vi "Measurement.WavelengthSweeping.GetStaticDependencies.vi"(8 "error in (no error)":errorcluster, 11 "Measurement.WavelengthSweeping in":refnum<class "Measurement.WavelengthSweeping.lvclass">) -> (0 "error out":errorcluster, 2 "Dependencies":T1, 3 "Measurement.WavelengthSweeping out":refnum<class "Measurement.WavelengthSweeping.lvclass">)   [LabVIEW 2019, in "Measurement.WavelengthSweeping.lvclass"]
uses:
  Measurement.WavelengthSweeping.lvclass
  C:/Program Files (x86)/National Instruments/LabVIEW 2019/vi.lib/JKI/JKI SMO/SMO/SMO.lvclass
  Typedefs/Dependencies--Cluster.ctl
  SMU/SMU.lvclass
  LIA/LIA.lvclass
  OPM/OPM.lvclass
  OPA/OPA.lvclass
  MC/MC.lvclass
  <vilib>/JKI/JKI SMO/SMO/SMO.lvclass
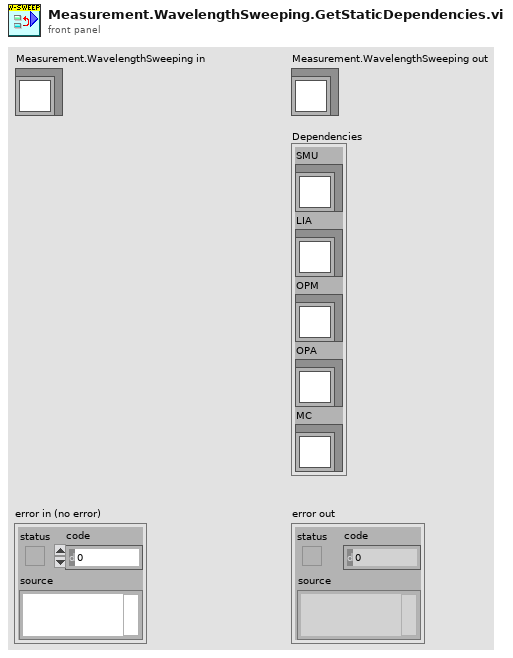
[diagram p1: front panel]
types:
  T1 = typedef "Measurement.WavelengthSweeping.lvclass/Dependencies--Cluster.ctl" = cluster{"SMU":refnum<class "SMU.lvclass">, "LIA":refnum<class "LIA.lvclass">, "OPM":refnum<class "OPM.lvclass">, "OPA":refnum<class "OPA.lvclass">, "MC":refnum<class "MC.lvclass">}
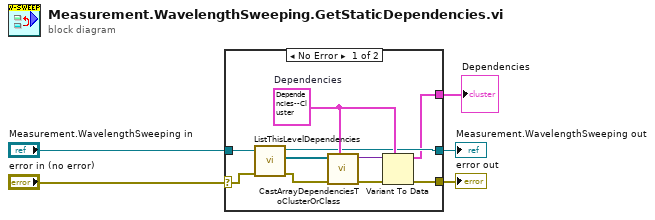
[diagram p0: block diagram]
diagram:
  n1 = case shown="No Error" "error in (no error)" {
    selector: "error in (no error)" -> [w14 w17]
    tunnel: [w8 w17] -> w4
    tunnel: [w7 w16] -> w2
    tunnel: "Measurement.WavelengthSweeping in" -> [w15 w16]
    tunnel: [w6 _] -> w1
    frame No Error {
      w9 = T1 {"SMU"=refnum, "LIA"=refnum, "OPM"=refnum, "OPA"=refnum, "MC"=refnum}  # Dependencies
      n2 = call <vilib>:"ListThisLevelDependencies.vi"("error in (no error)"=w14, "SMO in"=w15) -> ("error out"=w12:errorcluster, "[My Dependencies]"=w13:refnum<class "SMO.lvclass">[], "SMO out"=w7:refnum<class "Measurement.WavelengthSweeping.lvclass">)  [unwired: 7 in]
      n3 = call <vilib>:"CastArrayDependenciesToClusterOrClass.vi"("Dependency Type (Class|Cluster)"=w9, "error in (no error)"=w12, "[Dependencies]"=w13) -> ("error out"=w11:errorcluster, "Dependencies output"=w10:variant)  [unwired: 7 in]
      n4 = Variant To Data(error in=w11, type=w9, Variant=w10) -> (data=w6:T1, error out=w8:errorcluster)
    }
    frame Error {
    }
  }
  "error out" <- w4
  "Measurement.WavelengthSweeping out" <- w2
  "Dependencies" <- w1
